vi "Update Panel and Output State.vi"(3 "Events":refnum<vi>, 4 "DIO Panel reference":refnum<vi>, 5 "AD2":i32, 6 "Threshold panel reference":refnum<vi>, 7 "SG Device":T1(ring) caption="Signal Generator Device", 8 "error in":errorcluster, 9 "Use DIO":bool, 10 "Siglent Name":refnum<visa-resource-name>, 11 "Event name":T3) -> (0 "error out":errorcluster)   [LabVIEW 2024]
uses:
  Type Definitions/Threshold Events.ctl
  RT Core/Type Definitions/DIO_Cluster.ctl
  <instrlib>/Siglent SDG 1000 5000 800 Series/Siglent SDG 1000 5000 800 Series.lvlib
  Library/AD2/AD2 DLL.lvlib
panel:
  in  "DIO":T2
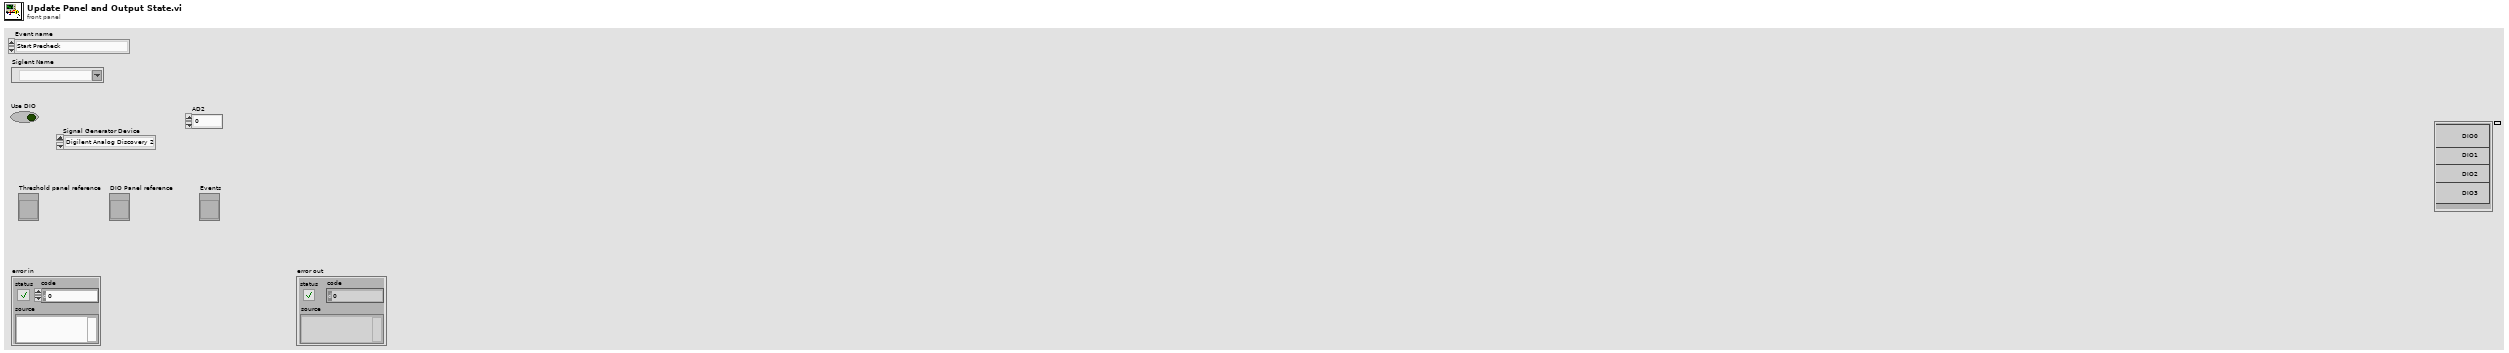
[diagram p1: front panel]
types:
  T1 = enum16{"Digilent Analog Discovery 2", "Siglent DG"}
  T2 = typedef "DIO_Cluster.ctl" = cluster{"DIO0":bool, "DIO1":bool, "DIO2":bool, "DIO3":bool}
  T3 = typedef "Threshold Events.ctl" = enum16{"Start Precheck", "Start Scenario", "Start Releasing", "Finish Releasing", "Clear Scenario", "Abort Scenario"}
  T4 = enum8{"Enabled", "Disabled", "Disabled and Grayed Out"}
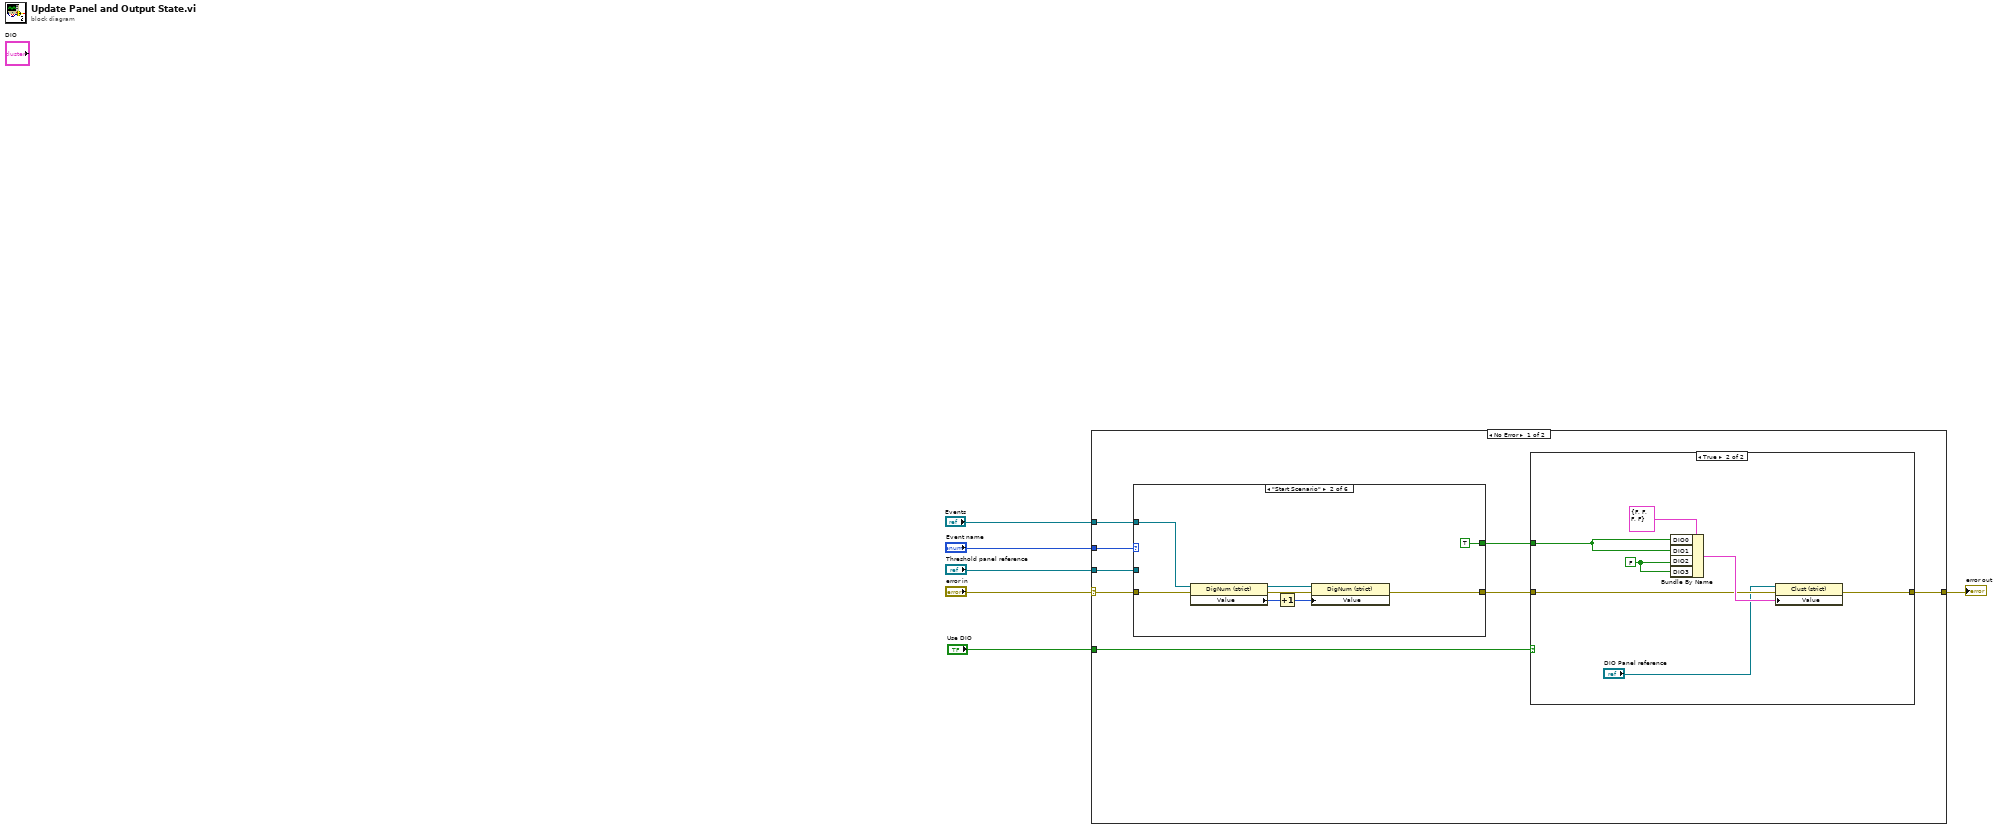
[diagram p0: block diagram]
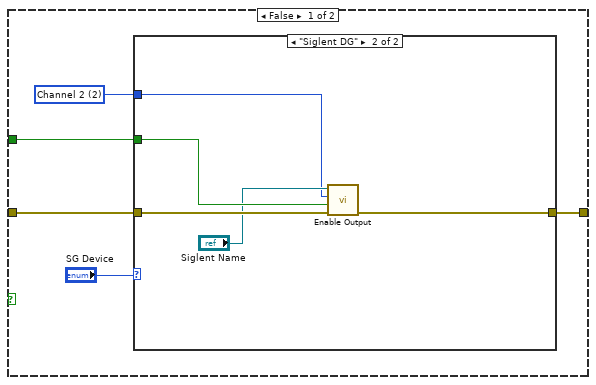
[diagram p2: hidden frame]
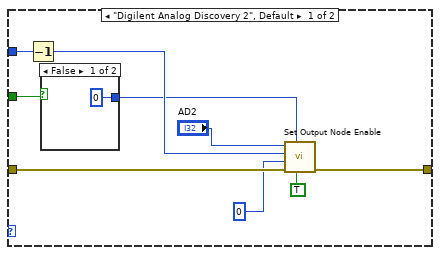
[diagram p3: hidden frame]
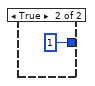
[diagram p4: hidden frame]
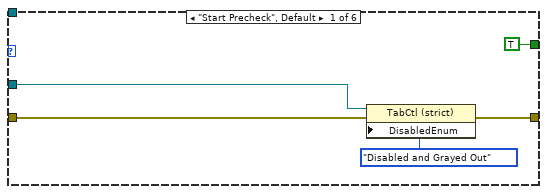
[diagram p5: hidden frame]
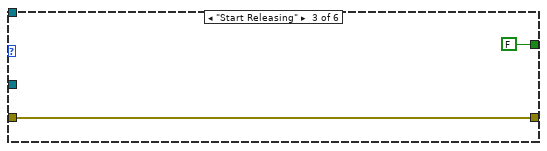
[diagram p6: hidden frame]
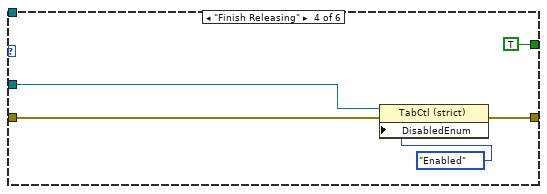
[diagram p7: hidden frame]
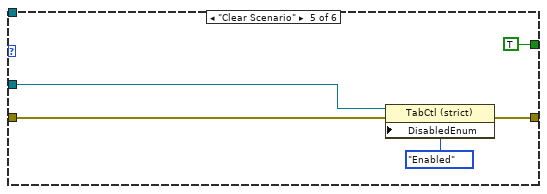
[diagram p8: hidden frame]
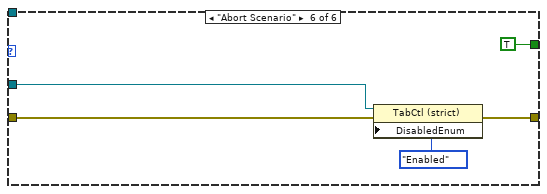
[diagram p9: hidden frame]
diagram:
  n1 = case shown="No Error" "error in" {
    selector: "error in" -> [w8 w73]
    tunnel: "Event name" -> [w14 _]
    tunnel: "Threshold panel reference" -> [w13 _]
    tunnel: [w11 w73] -> w4
    tunnel: "Use DIO" -> [w9 _]
    tunnel: "Events" -> [w7 _]
    frame No Error {
      n2 = case shown="\"Start Scenario\"" w14 {
        tunnel: w8 -> [w46 w54 w57 w60 w66 w71]
        tunnel: [w45 w51 w57 w59 w65 w70] -> w12
        tunnel: [TRUE TRUE FALSE TRUE TRUE TRUE] -> w10
        tunnel: w13 -> [w43 _ _ w58 w63 w68]
        tunnel: w7 -> [_ w53 _ _ _ _]
        frame "Start Precheck", Default {
          n3 = property on="Property Node" class="TabCtl (strict)"(reference=w43, error in=w46, "DisabledEnum"=T4."Disabled and Grayed Out" ("Disabled")) -> (error out=w45:errorcluster)  [unwired: 1 out]
        }
        frame "Start Scenario" {
          n4 = property class="DigNum (strict)"(reference=w53, error in=w54) -> (reference out=w50:refnum<vi>, error out=w52:errorcluster, "Value"=w49:i16)
          n5 = Increment(x=w49) -> (x+1=w48:i16)
          n6 = property class="DigNum (strict)"(reference=w50, error in=w52, "Value"=w48) -> (error out=w51:errorcluster)  [unwired: 1 out]
        }
        frame "Start Releasing" {
        }
        frame "Finish Releasing" {
          n7 = property on="Property Node" class="TabCtl (strict)"(reference=w58, error in=w60, "DisabledEnum"=T4."Enabled" ("Disabled")) -> (error out=w59:errorcluster)  [unwired: 1 out]
        }
        frame "Clear Scenario" {
          n8 = property on="Property Node" class="TabCtl (strict)"(reference=w63, error in=w66, "DisabledEnum"=T4."Enabled" ("Disabled")) -> (error out=w65:errorcluster)  [unwired: 1 out]
        }
        frame "Abort Scenario" {
          n9 = property on="Property Node" class="TabCtl (strict)"(reference=w68, error in=w71, "DisabledEnum"=T4."Enabled" ("Disabled")) -> (error out=w70:errorcluster)  [unwired: 1 out]
        }
      }
      n10 = case shown="True" w9 {
        tunnel: w12 -> [w19 w38]
        tunnel: [w18 w37] -> w11
        tunnel: w10 -> [w17 w40]
        frame False {
          w15 = 2 items=["Channel 1"=1, "Channel 2"=2] ("Channel (1:Channel 1)")
          n11 = case shown="\"Siglent DG\"" "SG Device" {
            tunnel: w19 -> [w25 w35]
            tunnel: [w24 w34] -> w18
            tunnel: w17 -> [w21 w33]
            tunnel: w15 -> [w28 w31]
            frame "Digilent Analog Discovery 2", Default {
              n12 = Decrement(x=w28) -> (x-1=w26:i32)
              n13 = case shown="False" w21 {
                tunnel: [0 ("Enable") 1 ("Enable")] -> w20
                frame False {
                }
                frame True {
                }
              }
              n14 = call "Set Output Node Enable.vi"("Update"=TRUE, "Enable"=w20, "error in (no error)"=w25, "node"=0, "idxChannel"=w26, "hdwf"="AD2") -> ("error out"=w24:errorcluster)  [unwired: 4 in, 1 out]
            }
            frame "Siglent DG" {
              n15 = call <instrlib>:"Enable Output.vi"("error in (no error)"=w35, "Enable Output (T: Enable)"=w33, "Channel (1:Channel 1)"=w31, "VISA resource name"="Siglent Name") -> ("error out"=w34:errorcluster)  [unwired: 6 in, 1 out]
            }
          }
        }
        frame True {
          w41 = FALSE
          n16 = Bundle By Name(cluster=T2 {"DIO0"=FALSE, "DIO1"=FALSE, "DIO2"=FALSE, "DIO3"=FALSE} ("DIO"), "DIO0"=w40, "DIO1"=w40, "DIO2"=w41, "DIO3"=w41) -> (w39:T2)
          n17 = property on="Property Node" class="Clust (strict)"(reference="DIO Panel reference", error in=w38, "Value"=w39) -> (error out=w37:errorcluster)  [unwired: 1 out]
        }
      }
    }
    frame Error {
    }
  }
  "error out" <- w4
